vi "Model_statues.vi"(8 "error in (no error)":errorcluster caption="错误输入（无错误）", 11 "User Management Model 输入":refnum<class "User Management Model.lvclass">) -> (0 "error out":errorcluster caption="错误输出", 2 "用户信息":T1, 3 "User Management Model 输出":refnum<class "User Management Model.lvclass">)   [LabVIEW 2019, in "User Management Model.lvclass"]
uses:
  User Management Model.lvclass
  protect/ObjectAttributes.ctl
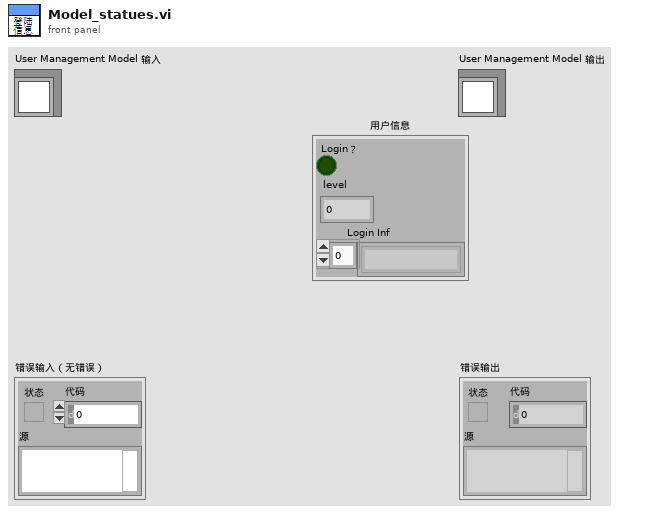
[diagram p1: front panel]
types:
  T1 = typedef "User Management Model.lvclass/ObjectAttributes.ctl" = cluster{"Login？":bool, "level":i32, "Login Inf":string[]}
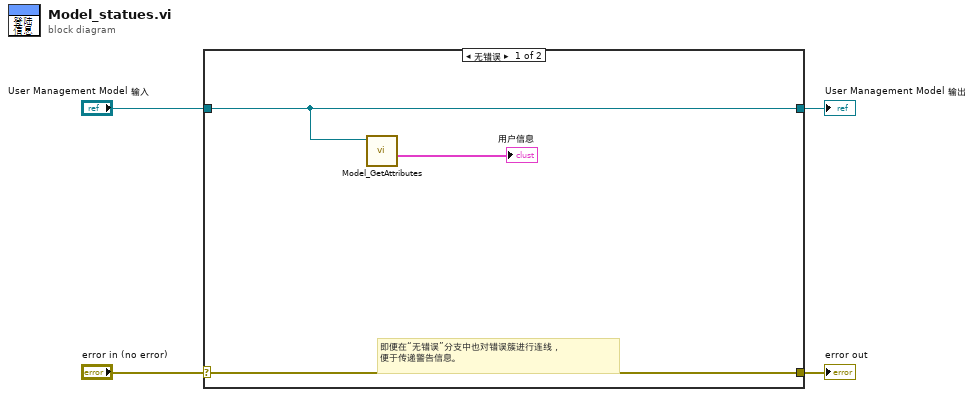
[diagram p0: block diagram]
diagram:
  n1 = case shown="无错误" "error in (no error)" {
    selector: "error in (no error)" -> [w7 w9]
    tunnel: [w7 w9] -> w3
    tunnel: [w6 w8] -> w1
    tunnel: "User Management Model 输入" -> [w6 w8]
    frame No Error {
      # "即便在“无错误”分支中也对错误簇进行连线，\n便于传递警告信息。"
      n2 = call "Model_GetAttributes.vi"("User Management Model 输入"=w6) -> ("数据值"=→"用户信息":T1)  [unwired: 7 in, 3 out]
    }
    frame Error {
    }
  }
  "error out" <- w3
  "User Management Model 输出" <- w1
